vi "SetButtonControls.vi"(8 "ErrorIn":errorcluster caption="Error In", 9 "Buttons":refnum<vi>[](array[refnum]), 11 "ObjectIn":refnum<class "ButtonCollection.lvclass"> caption="Object In") -> (0 "ErrorOut":errorcluster caption="Error Out", 3 "ObjectOut":refnum<class "ButtonCollection.lvclass"> caption="Object Out")   [LabVIEW 2021, in "ButtonCollection.lvclass"]
uses:
  ButtonCollection.lvclass
  ButtonCollection.lvclass/ButtonCollection.ctl
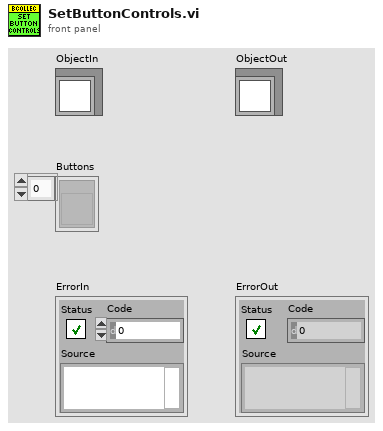
[diagram p1: front panel]
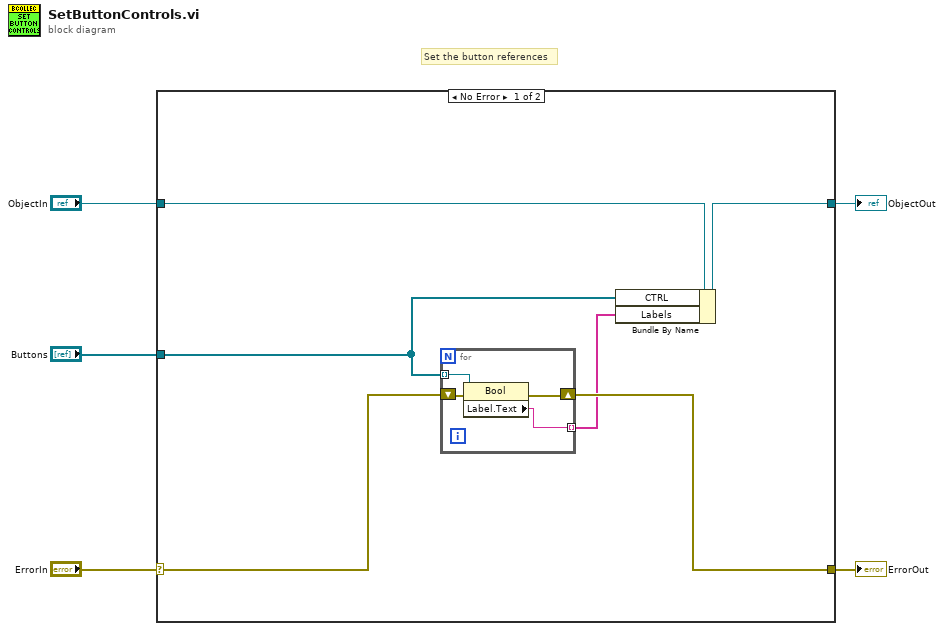
[diagram p0: block diagram]
diagram:
  # "Set the button references"
  n1 = case shown="No Error" "ErrorIn" {
    selector: "ErrorIn" -> [w11 w17]
    tunnel: [w10 w17] -> w4
    tunnel: [w8 w16] -> w2
    tunnel: "ObjectIn" -> [w9 w16]
    tunnel: "Buttons" -> [w7 _]
    frame No Error {
      n2 = for {
        tunnel: w7 -> [w13] mode=indexing
        tunnel: [w12] -> w6 mode=indexing
        shift-right: [w14] -> w10
        shift-left: w11 -> [w15]
        n3 = property class="Bool"(reference=w13, error in=w15) -> (error out=w14:errorcluster, "Label.Text"=w12:string)  [unwired: 1 out]
      }
      n4 = Bundle By Name(cluster=w9, "CTRL"=w7, "Labels"=w6) -> (w8:refnum<class "ButtonCollection.lvclass">)
    }
    frame Error {
    }
  }
  "ErrorOut" <- w4
  "ObjectOut" <- w2
